vi "EnableControlSub.vi"(0 "dt":dbl, 1 "Torque":bool, 2 "ResetAngle":dbl, 3 "复位速率":dbl=0.999 format="%#_13g", 5 "TorqueSample0":dbl, 7 "Angel":bool, 9 "AngleSample0":dbl, 11 "ChannelStatus":T1 items=["通道关", "位置通道", "加载通道"], 12 "ResetTorque":dbl, 13 "output range":cluster{"output high":dbl, "output low":dbl}={"output high"=2.0, "output low"=-2.0}, 14 "簇":cluster{dbl, dbl, dbl}) -> (4 "ResetTorque 2":dbl, 6 "ResetAngle 2":dbl, 10 "ControlOutput":dbl, 15 "Commandout":dbl)   [LabVIEW 2014]
uses:
  Control 1.ctl
  <vilib>/addons/control/pid/pid.llb/PID (DBL).vi
  <vilib>/addons/control/pid/NI_PID_pid.lvlib
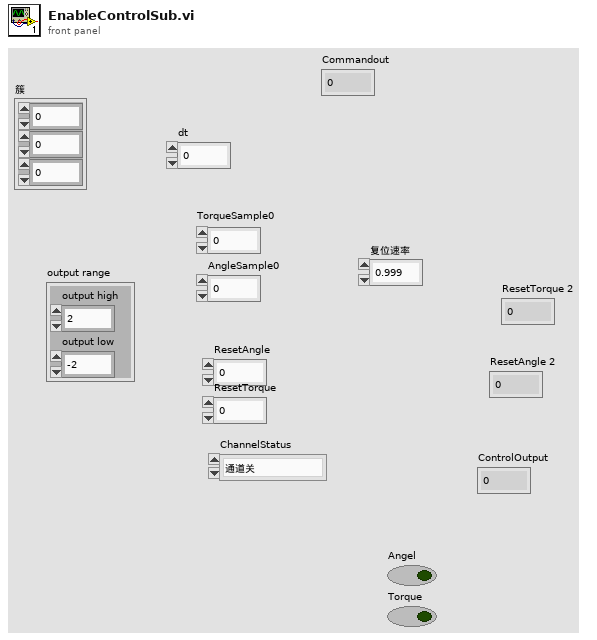
[diagram p1: front panel]
types:
  T1 = typedef "Control 1.ctl" = i32
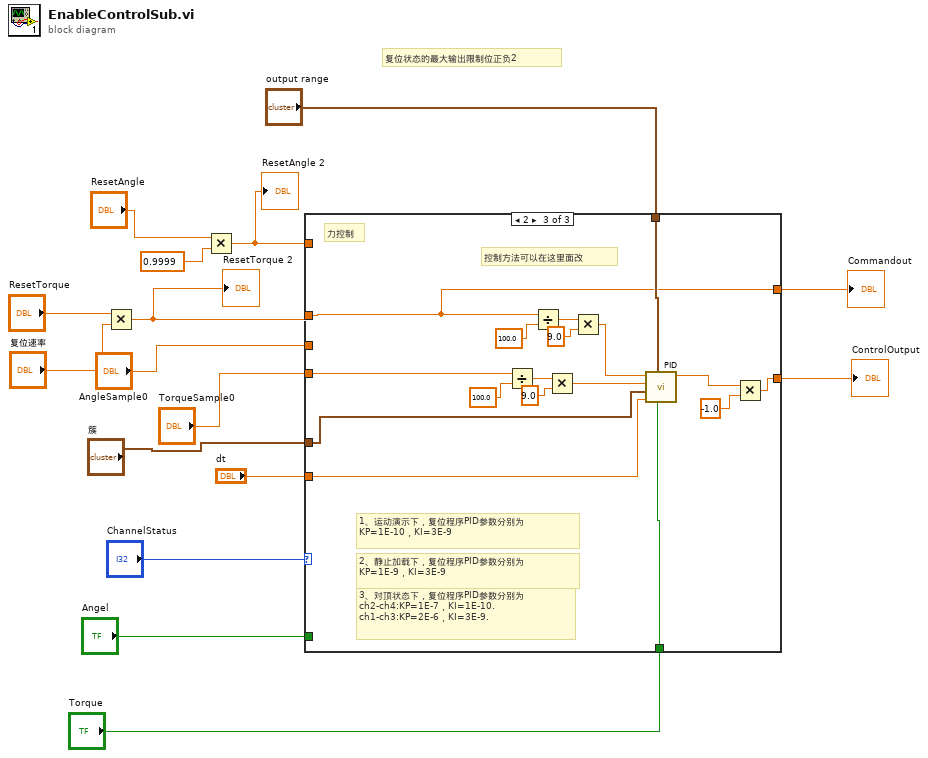
[diagram p0: block diagram]
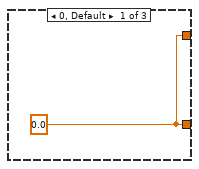
[diagram p2: hidden frame]
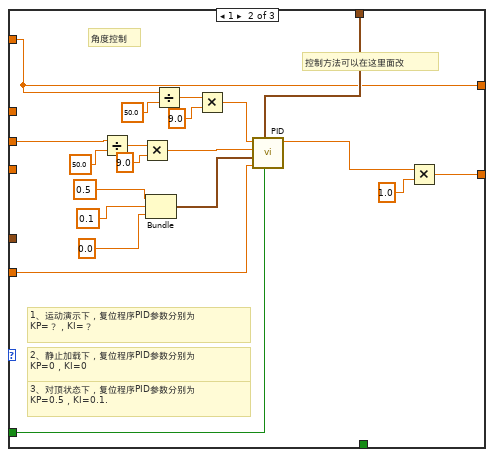
[diagram p3: hidden frame]
diagram:
  # "复位状态的最大输出限制位正负2"
  n1 = Multiply(x="ResetTorque", y="复位速率") -> (x*y=w11:dbl)
  "ResetTorque 2" <- w11
  n2 = Multiply(x="ResetAngle", y=0.9999) -> (x*y=w10:dbl)
  "ResetAngle 2" <- w10
  n3 = case shown="2" "ChannelStatus" {
    tunnel: "dt" -> [_ w37 w54]
    tunnel: [w17 w21 w44] -> w5
    tunnel: "output range" -> [_ w36 w53]
    tunnel: w11 -> [_ _ w40]
    tunnel: w10 -> [_ w18 _]
    tunnel: "TorqueSample0" -> [_ _ w42]
    tunnel: "AngleSample0" -> [_ w20 _]
    tunnel: "Angel" -> [_ w19 _]
    tunnel: "Torque" -> [_ _ w41]
    tunnel: [w17 w18 w40] -> w2
    tunnel: "簇" -> [_ _ w38]
    frame 0, Default {
      w17 = 0.0 ("output")
    }
    frame 1 {
      # "1、运动演示下，复位程序PID参数分别为\nKP=？，KI=？"
      # "2、静止加载下，复位程序PID参数分别为\nKP=0，KI=0"
      # "3、对顶状态下，复位程序PID参数分别为\nKP=0.5，KI=0.1."
      # "控制方法可以在这里面改"
      # "角度控制"
      n4 = Divide(x=w20, y=50.0) -> (x/y=w32:dbl)
      n5 = Multiply(x=w32, y=9.0) -> (x*y=w31:dbl)
      n6 = Bundle(0.5, 0.1, 0.0) -> (w35:cluster{dbl, dbl, dbl})  [unwired: 1 in]
      n7 = Divide(x=w18, y=50.0) -> (x/y=w28:dbl)
      n8 = Multiply(x=w28, y=9.0) -> (x*y=w27:dbl)
      n9 = call-poly <vilib>:"PID.vi"("reinitialize? (F)"=w19, "output range"=w36, "dt (s)"=w37, "PID gains"=w35, "process variable"=w31, "setpoint"=w27) -> ("output"=w25:dbl)  [unwired: 4 in, 1 out]
      n10 = Multiply(x=w25, y=1.0) -> (x*y=w21:dbl)
    }
    frame 2 {
      # "1、运动演示下，复位程序PID参数分别为\nKP=1E-10，KI=3E-9"
      # "2、静止加载下，复位程序PID参数分别为\nKP=1E-9，KI=3E-9"
      # "3、对顶状态下，复位程序PID参数分别为\nch2-ch4:KP=1E-7，KI=1E-10. \nch1-ch3:KP=2E-6，KI=3E-9."
      # "力控制"
      # "控制方法可以在这里面改"
      n11 = Divide(x=w42, y=100.0) -> (x/y=w46:dbl)
      n12 = Divide(x=w40, y=100.0) -> (x/y=w50:dbl)
      n13 = Multiply(x=w46, y=9.0) -> (x*y=w45:dbl)
      n14 = Multiply(x=w50, y=9.0) -> (x*y=w49:dbl)
      n15 = call-poly <vilib>:"PID.vi"("reinitialize? (F)"=w41, "output range"=w53, "dt (s)"=w54, "PID gains"=w38, "process variable"=w45, "setpoint"=w49) -> ("output"=w43:dbl)  [unwired: 4 in, 1 out]
      n16 = Multiply(x=w43, y=-1.0) -> (x*y=w44:dbl)
    }
  }
  "ControlOutput" <- w5
  "Commandout" <- w2
